vi "RESIDUALdll.vi"(8 "error in (no error)":errorcluster, 11 "Inputs":cluster{"t":dbl, "D":dbl, "z":dbl[]}) -> (0 "error out":errorcluster, 3 "Outputs":T1)   [LabVIEW 2021]
doc: "subroutine RESIDUALdll(t, d, z, pr, er, hr, sr, cvr, cpr, ar, gr)\n\nCompute the residual quantities as a function of temperature, density,\nand compositions (where the residual is the property minus the ideal\ngas portion).\n\nINPUTS:\nt -- temperature [K]\nD -- molar density [mol/L]\nz -- composition [array of mol frac]\n\nOUTPUTS:\npr -- residual pressure [kPa] (p-rho*R*T)\ner -- residual internal energy [J/mol]\nhr -- residual enthalpy [J/mol]\nsr -- residual entropy [J/mol-K]\ncvr -- residual isochoric heat capacity [J/mol-K]\ncpr -- residual isobaric heat capacity [J/mol-K]\nar -- residual Helmholtz energy [J/mol]\ngr -- residual Gibbs free energy [J/mol]"
uses:
  REFPROP.dll
panel:
  # "REFPROP-RESIDUALdll.vi"
  # "void  RESIDUALdll(double *t, double *D, double *z, double *pr, double *er, double *hr, double *sr, double *cvr, double *cpr, double *ar, double *gr)"
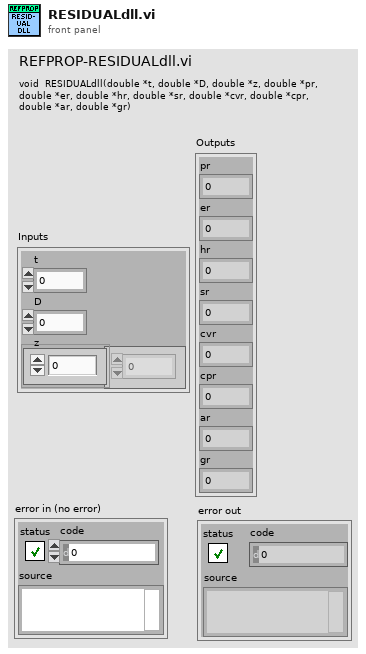
[diagram p1: front panel]
types:
  T1 = cluster{"pr":dbl, "er":dbl, "hr":dbl, "sr":dbl, "cvr":dbl, "cpr":dbl, "ar":dbl, "gr":dbl}
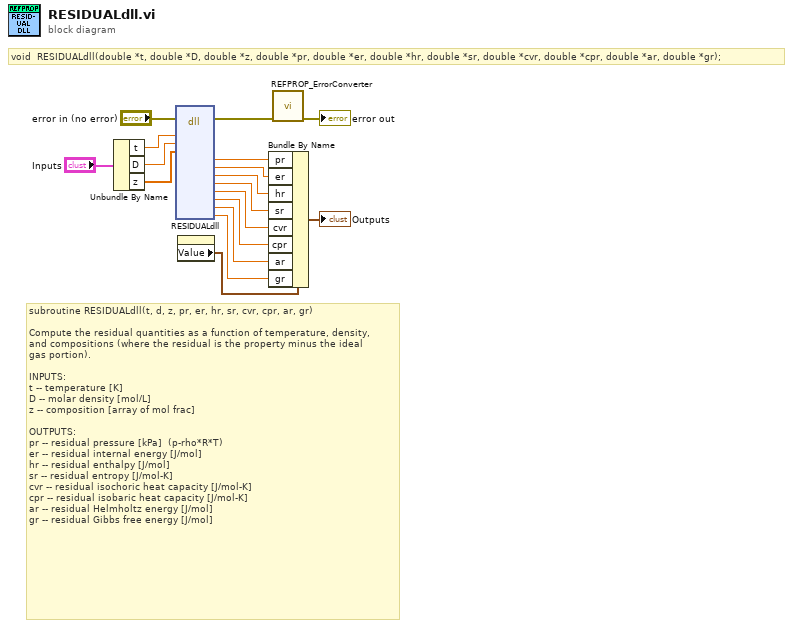
[diagram p0: block diagram]
diagram:
  # "void  RESIDUALdll(double *t, double *D, double *z, double *pr, double *er, double *hr, double *sr, double *cvr, double *cpr, double *ar, double *gr);"
  # "subroutine RESIDUALdll(t, d, z, pr, er, hr, sr, cvr, cpr, ar, gr)\n\nCompute the residual quantities as a function of temperature, density,\nand compositions (where the residual is the property minus the ideal\ngas portion).\n\nINPUTS:\nt -- temperature [K]\nD -- molar density [mol/L]\nz -- composition [array of mol frac]\n\nOUTPUTS:\npr -- residual pressure [kPa]  (p-rho*R*T)\ner -- residual internal energy [J/mol]\nhr -- residual enthalpy [J/mol]\nsr -- residual entropy [J/mol-K]\ncvr -- residual isochoric heat capacity [J/mol-K]\ncpr -- residual isobaric heat capacity [J/mol-K]\nar -- residual Helmholtz energy [J/mol]\ngr -- residual Gibbs free energy [J/mol]"
  n1 = Unbundle By Name("Inputs") -> ("t"=w13:dbl, "D"=w12:dbl, "z"=w11:dbl[])
  n2 = dll-call lib="C:/Users/lauria/OneDrive - National Institute of Standards and Technology (NIST)/LabVIEW Projects/7 REFPROP/REFPROP-wrappers-master/REFPROP-wrappers-master/wrappers/Labview/REFPROP/REFPROP.*" fn="RESIDUALdll"(error in="error in (no error)", "t"=w13, "D"=w12, "z"=w11) -> (error out=w17:errorcluster, "pr"=w9:dbl, "er"=w7:dbl, "hr"=w6:dbl, "sr"=w5:dbl, "cvr"=w4:dbl, "cpr"=w3:dbl, "ar"=w2:dbl, "gr"=w1:dbl)  [unwired: 14 in, 1 out]
  n3 = property on="Outputs" class="Clust (strict)"() -> ("Value"=w8:T1)  [unwired: 2 in, 2 out]
  n4 = Bundle By Name(cluster=w8, "pr"=w9, "er"=w7, "hr"=w6, "sr"=w5, "cvr"=w4, "cpr"=w3, "ar"=w2, "gr"=w1) -> (→"Outputs":T1)
  n5 = call "REFPROP_ErrorConverter.vi"("error in (no error)"=w17) -> ("error out"=→"error out":errorcluster)  [unwired: 10 in]
